vi "main2.vi"() -> ()   [LabVIEW 2014]
panel:
  in  "탭 컨트롤":enum32{"Setting", "Test"}(tab)
  out "웨이브폼 차트":dbl(graph)
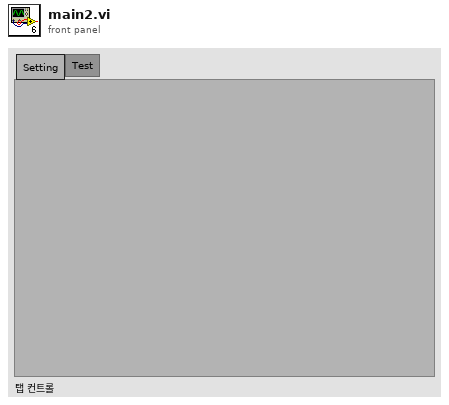
[diagram p1: front panel]
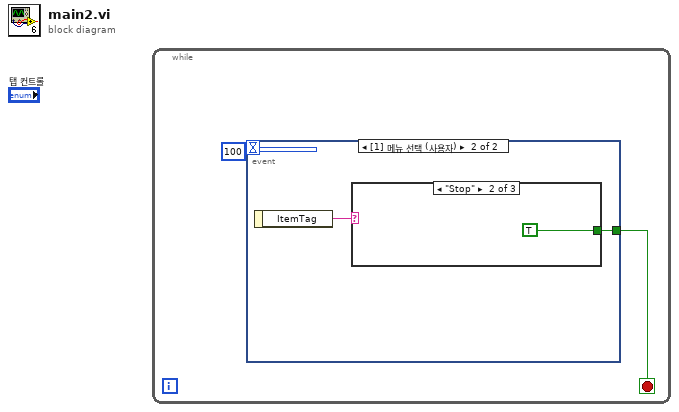
[diagram p0: block diagram]
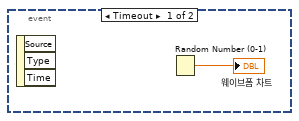
[diagram p2: hidden frame]
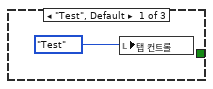
[diagram p3: hidden frame]
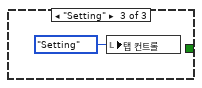
[diagram p4: hidden frame]
diagram:
  n1 = while {
    stop <- w1 stop-if-true
    n2 = event shown="[1] 메뉴 선택 (사용자)" {
      selector: _ -> [_ _]
      dyn-events: _ -> [_ _]
      timeout: 100 -> [_ _]
      tunnel: [_ w4] -> w1
      event Timeout {
        n3 = event-data() -> ()  [unwired: 1 in, 3 out]
        n4 = Random Number (0-1)() -> (number: 0 to 1=→"웨이브폼 차트":dbl)
      }
      event Menu Selection (User) {
        n5 = event-data() -> ("ItemTag"=w5:string)  [unwired: 1 in]
        n6 = case shown="\"Stop\"" w5 {
          tunnel: [_ TRUE _] -> w4
          frame "Test", Default {
            n7 = local write "탭 컨트롤"(enum32{"Setting", "Test"}."Test" ("탭 컨트롤")) -> ()
          }
          frame "Stop" {
          }
          frame "Setting" {
            n8 = local write "탭 컨트롤"(enum32{"Setting", "Test"}."Setting" ("탭 컨트롤")) -> ()
          }
        }
      }
    }
  }
